vi "Scan_Table_Mode.vi"(1 "Mode":T1) -> (0 "Simulate Mode ?":bool)   [LabVIEW 2010]
uses:
  Anemometry/Anemometry Sub Vis/Controls/Serveds.ctl
  Anemometry/Anemometry Sub Vis/Globals/Constants_global.vi
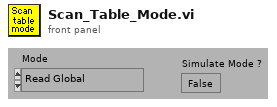
[diagram p1: front panel]
types:
  T1 = typedef "Serveds.ctl" = enum16{"Read Global", "Load Global From File"}
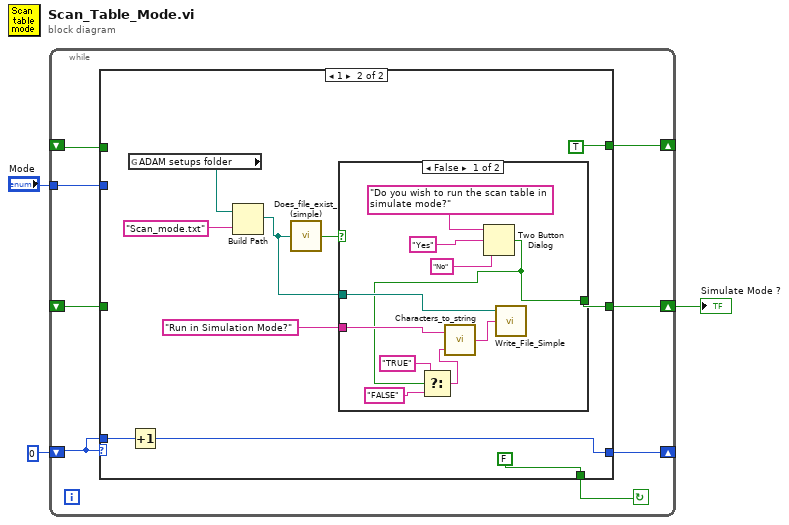
[diagram p0: block diagram]
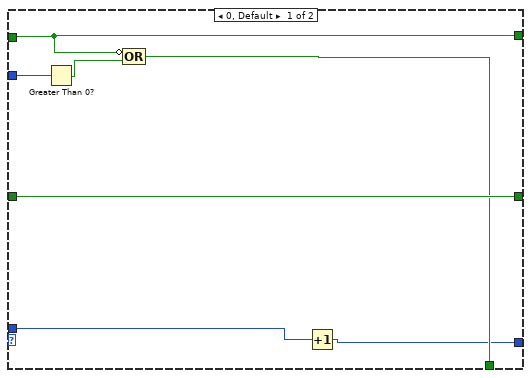
[diagram p2: hidden frame]
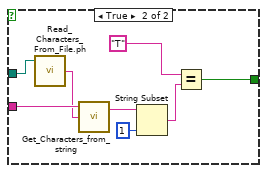
[diagram p3: hidden frame]
diagram:
  n1 = while {
    tunnel: "Mode" -> [w5]
    shift-left: 0 -> [w6]
    shift-right: [w8] -> _
    shift-left: _ -> [w10]
    shift-right: [w7] -> w1
    shift-left: _ -> [w11]
    shift-right: [w4] -> _
    stop <- w9 continue-if-true
    n2 = case shown="1" w6 {
      tunnel: w11 -> [w12 _]
      tunnel: w10 -> [w18 _]
      tunnel: [w15 FALSE] -> w9
      tunnel: [w13 w26] -> w8
      tunnel: [w18 w22] -> w7
      tunnel: w6 -> [w14 w27]
      tunnel: w5 -> [w17 _]
      tunnel: [w12 TRUE] -> w4
      frame 0, Default {
        n3 = Greater Than 0?(x=w17) -> (x > 0?=w16:bool)
        n4 = Compound Arithmetic op=OR(invert w12, w16) -> (w15:bool)
        n5 = Increment(x=w14) -> (x+1=w13:i32)
      }
      frame 1 {
        n6 = global read "Constants_global.vi" "ADAM setups folder"() -> (w25:path)
        n7 = Increment(x=w27) -> (x+1=w26:i32)
        n8 = Build Path(base path=w25, name or relative path="Scan_mode.txt" ("Substring")) -> (appended path=w20:path)
        n9 = call "Does_file_exist_(simple).vi"("Pathname"=w20) -> ("exists?"=w23:bool)
        n10 = case shown="False" w23 {
          tunnel: w20 -> [w37 w46]
          tunnel: [w29 w42] -> w22
          tunnel: "Run in Simulation Mode?" ("character string") -> [w38 w45]
          frame False {
            n11 = Two Button Dialog(message="Do you wish to run the scan table in simulate mode?", 1:"No" ("F button name (\"Cancel\")"), 2:"Yes" ("T button name (\"OK\")")) -> (T button?=w29:bool)
            n12 = Select(t="TRUE" ("Characters to write"), s=w29, f="FALSE") -> (s? t:f=w30:string)
            n13 = call "Characters_to_string.vi"("Characters to write"=w30, "Label for characters"=w38) -> ("Output string"=w36:string)
            n14 = call "Write_File_Simple.vi"("character string"=w36, "file path"=w37) -> ()  [unwired: 1 in, 2 out]
          }
          frame True {
            n15 = call "Read_Characters_From_File.ph.vi"("file path (dialog if empty)"=w46) -> ("character string"=w44:string)  [unwired: 1 in, 7 out]
            n16 = call "Get_Characters_from_string.vi"("Input string"=w44, "Variable name"=w45) -> ("Value"=w41:string)  [unwired: 1 in, 1 out]
            n17 = String Subset(string=w41, length (rest)=1 ("length (rest)")) -> (substring=w39:string)  [unwired: 1 out]
            n18 = Equal?(x="T", y=w39) -> (x = y?=w42:bool)
          }
        }
      }
    }
  }
  "Simulate Mode ?" <- w1
